vi "Main.vi"() -> ()   [LabVIEW 2017]
uses:
  support/Data Share Type.ctl
  D:/upwork/urartu project/urartu/vs/MapNetControl/bin/Debug/MapNetControl.dll
  vs/MapNetControl/bin/Debug/MapNetControl.dll
panel:
  in  "Add Button":bool
  in  "Longitude, deg:":dbl=27.559764
  in  "Latitude, deg:":dbl=53.907767
  in  "Map folder:":path
  in  "Exit Button":bool
  in  "MapNetControl":refnum<k24>(container)
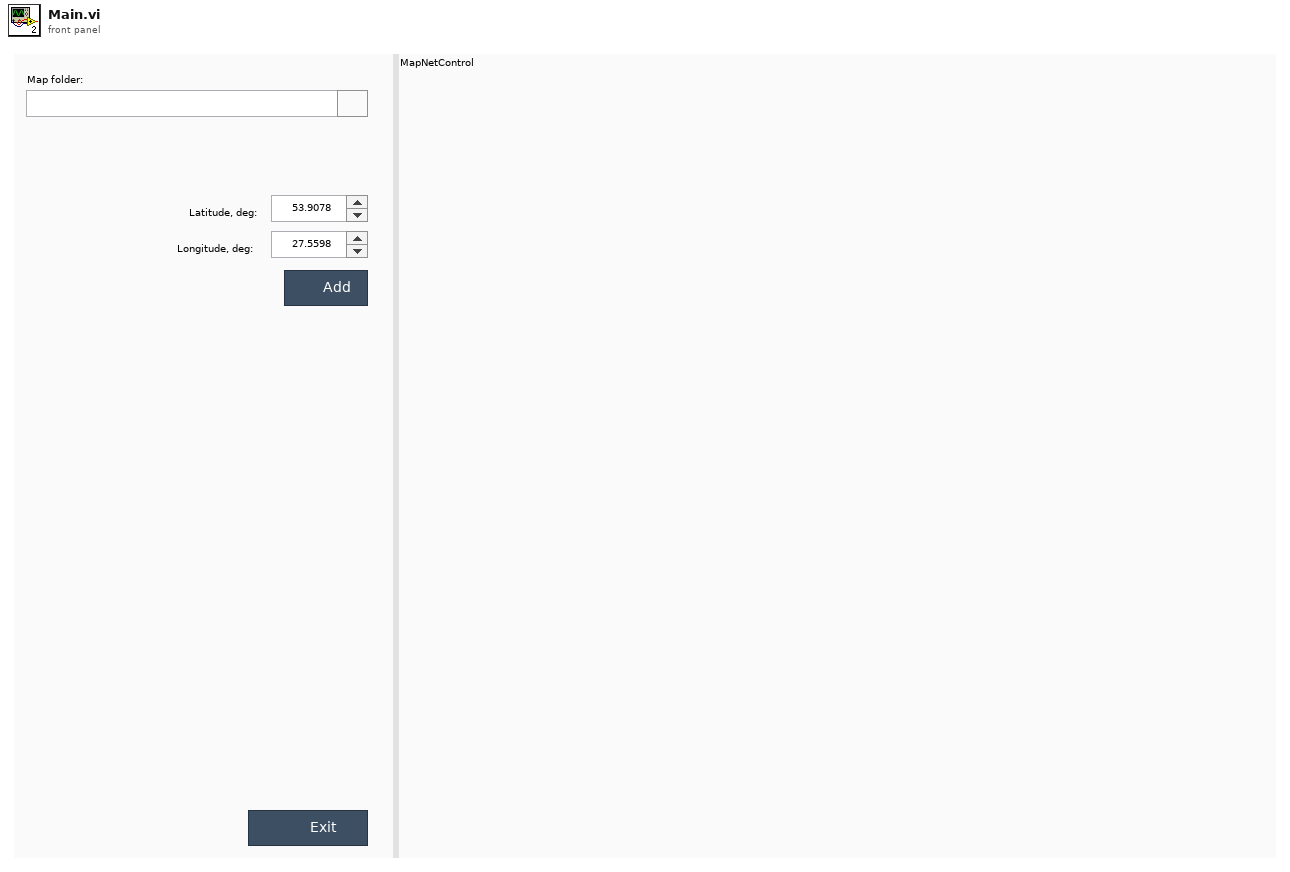
[diagram p1: front panel]
types:
  T1 = typedef "Data Share Type.ctl" = cluster{"Map folder":path, "Latitude, deg:":dbl, "Longitude, deg:":dbl}
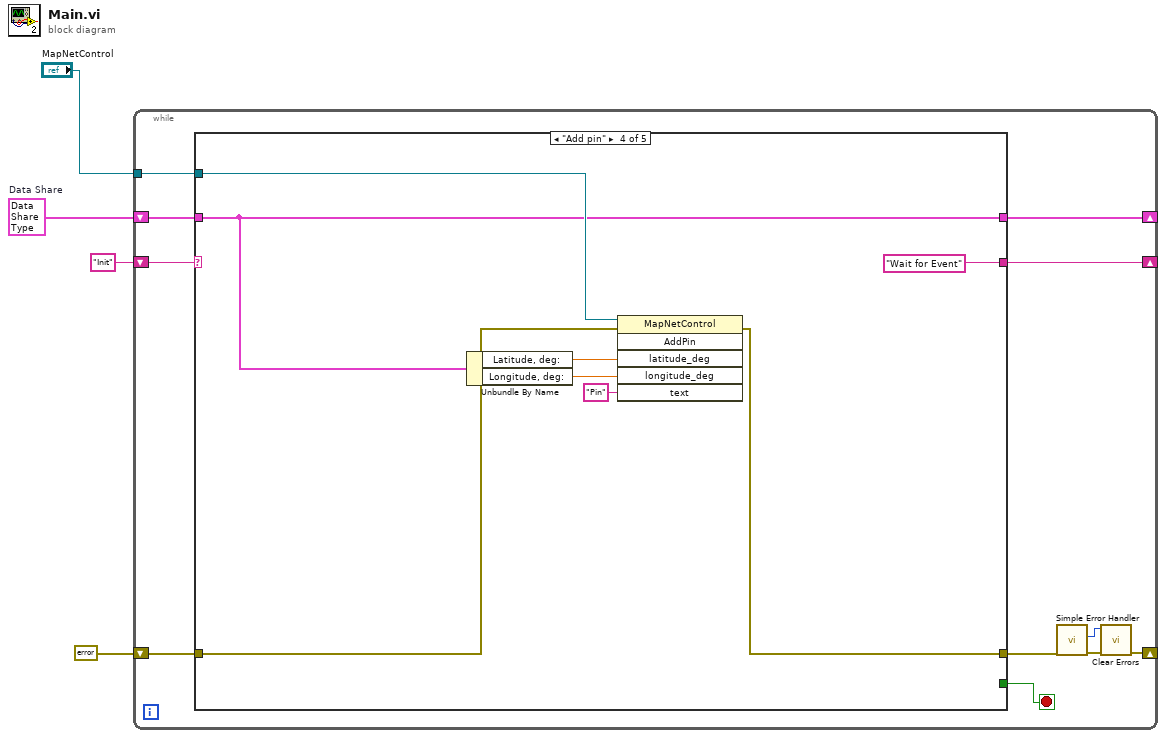
[diagram p0: block diagram]
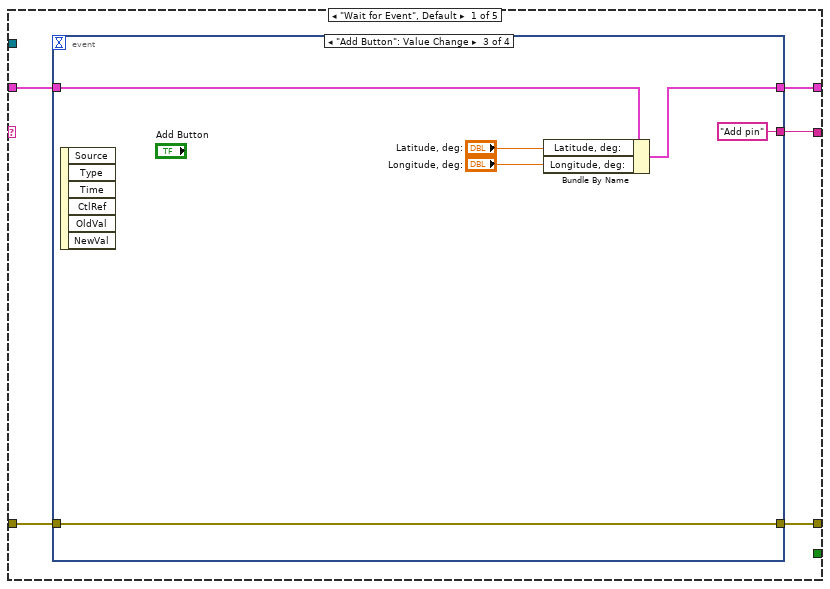
[diagram p2: hidden frame]
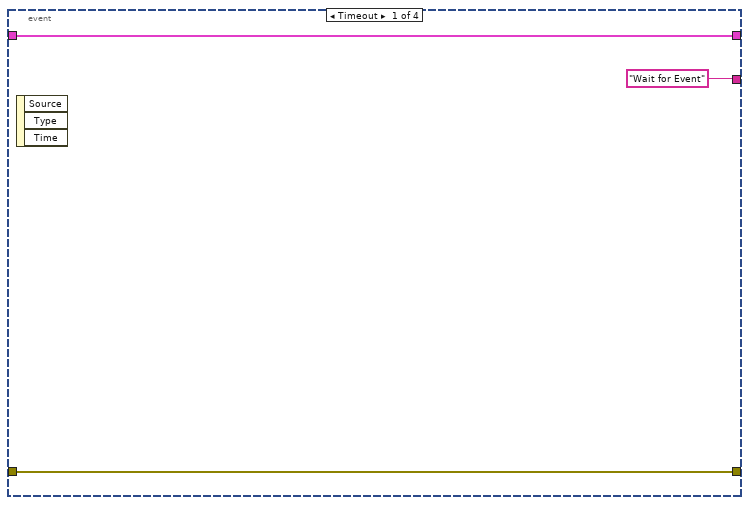
[diagram p3: hidden frame]
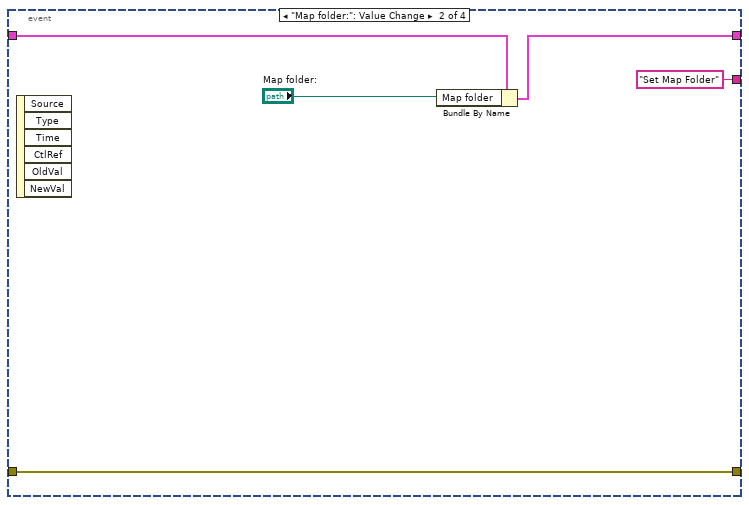
[diagram p4: hidden frame]
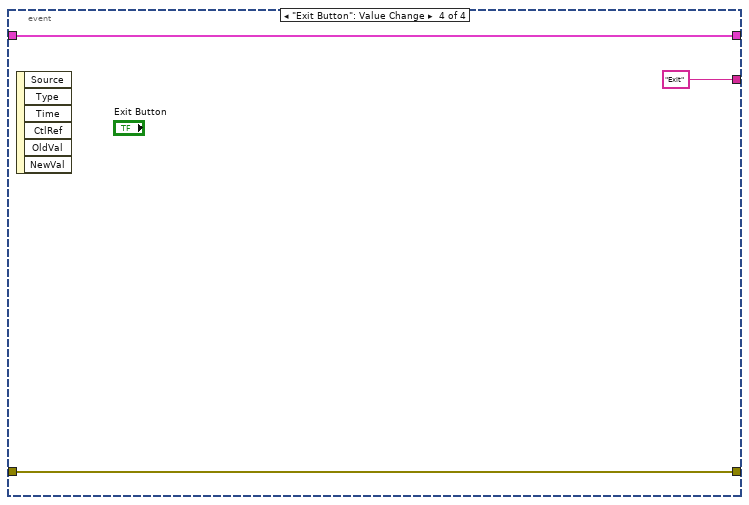
[diagram p5: hidden frame]
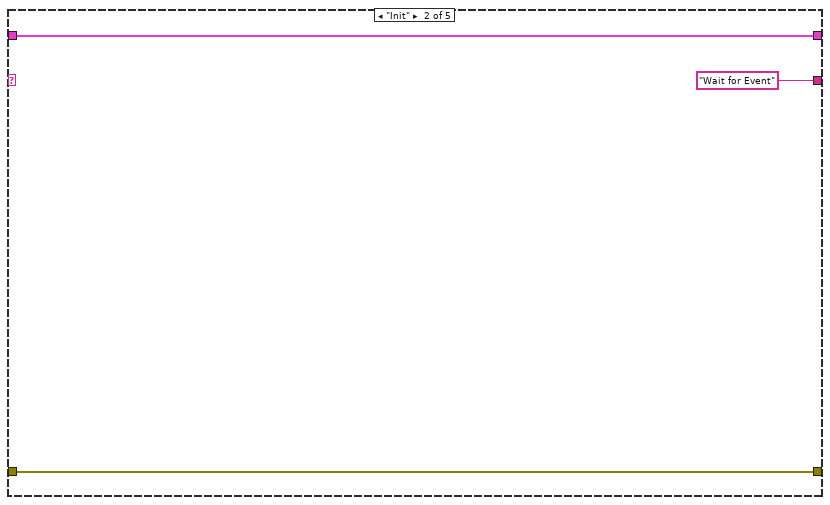
[diagram p6: hidden frame]
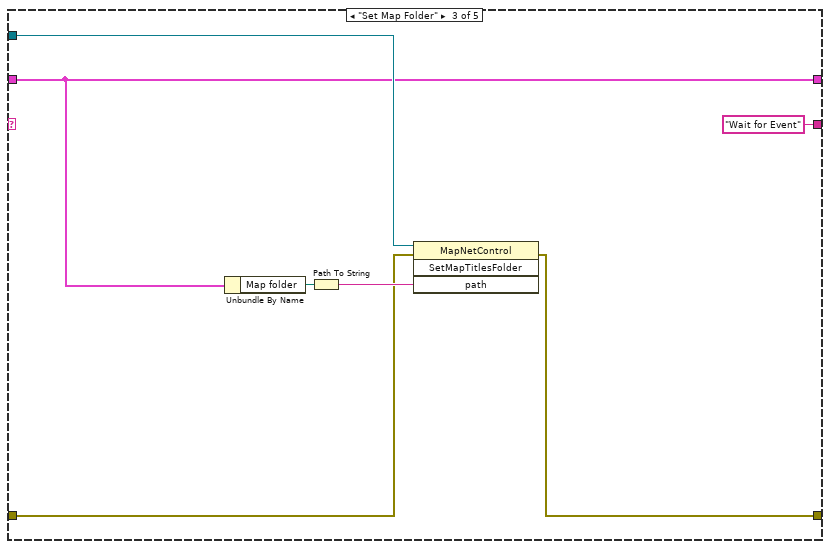
[diagram p7: hidden frame]
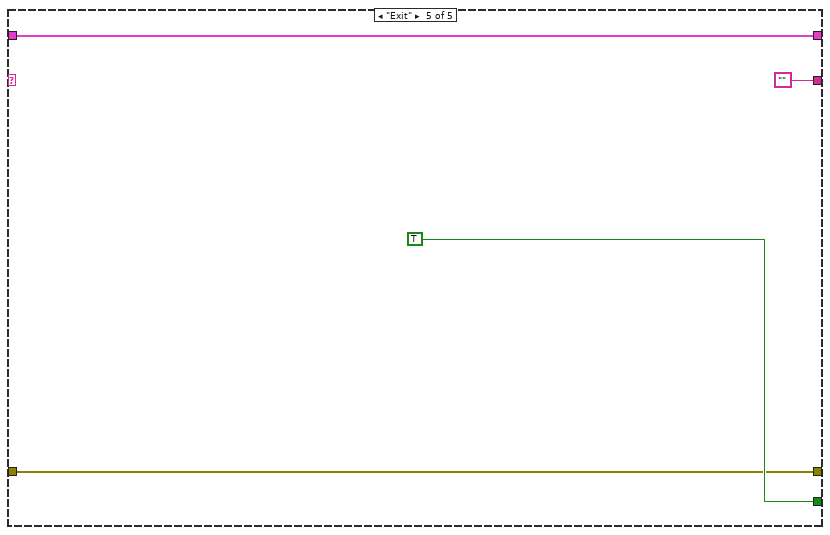
[diagram p8: hidden frame]
diagram:
  w2 = T1 {"Map folder"=path "", "Latitude, deg:"=53.907767, "Longitude, deg:"=27.559764}  # Data Share
  n1 = while {
    tunnel: "MapNetControl" -> [w12]
    shift-right: [w14] -> _
    shift-left: "Init" -> [w15]
    shift-right: [w10] -> _
    shift-left: w2 -> [w11]
    shift-right: [w5] -> _
    shift-left: errorcluster {"status"=FALSE, "code"=0, "source"=""} ("error in (no error)") -> [w9]
    stop <- w13 stop-if-true
    n2 = case shown="\"Add pin\"" w15 {
      tunnel: [w20 "Wait for Event" "Wait for Event" "Wait for Event" ""] -> w14
      tunnel: [_ _ _ _ TRUE] -> w13
      tunnel: w12 -> [_ _ w45 w54 _]
      tunnel: w11 -> [w19 w39 w44 w51 w57]
      tunnel: [w18 w39 w44 w51 w57] -> w10
      tunnel: w9 -> [w17 w38 w42 w53 w56]
      tunnel: [w16 w38 w41 w52 w56] -> w8
      frame "Wait for Event", Default {
        n3 = event shown="[2] \"Add Button\": Value Change" {
          selector: _ -> [_ _ _ _]
          dyn-events: _ -> [_ _ _ _]
          timeout: _ -> [_ _ _ _]
          tunnel: ["Wait for Event" "Set Map Folder" "Add pin" "Exit"] -> w20
          tunnel: [w22 w27 w31 w36] -> w18
          tunnel: w19 -> [w22 w28 w32 w36]
          tunnel: w17 -> [w21 w24 w34 w35]
          tunnel: [w21 w24 w34 w35] -> w16
          event Timeout {
            n4 = event-data() -> ()  [unwired: 1 in, 3 out]
          }
          event "Map folder:": Value Change {
            n5 = event-data() -> ()  [unwired: 1 in, 6 out]
            n6 = Bundle By Name(cluster=w28, "Map folder"="Map folder:") -> (w27:T1)
          }
          event "Add Button": Value Change {
            n7 = event-data() -> ()  [unwired: 1 in, 6 out]
            n8 = Bundle By Name(cluster=w32, "Latitude, deg:"="Latitude, deg:", "Longitude, deg:"="Longitude, deg:") -> (w31:T1)
          }
          event "Exit Button": Value Change {
            n9 = event-data() -> ()  [unwired: 1 in, 6 out]
          }
        }
      }
      frame "Init" {
      }
      frame "Set Map Folder" {
        n10 = Unbundle By Name(w44) -> ("Map folder"=w43:path)
        n11 = Path To String(path=w43) -> (string=w46:string)
        n12 = invoke class="MapNetControl" method="SetMapTitlesFolder"(reference=w45, error in=w42, "path"=w46) -> (error out=w41:errorcluster)  [unwired: 1 in, 3 out]
      }
      frame "Add pin" {
        n13 = Unbundle By Name(w51) -> ("Latitude, deg:"=w50:dbl, "Longitude, deg:"=w49:dbl)
        n14 = invoke class="MapNetControl" method="AddPin"(reference=w54, error in=w53, "latitude_deg"=w50, "longitude_deg"=w49, "text"="Pin") -> (error out=w52:errorcluster)  [unwired: 1 in, 5 out]
      }
      frame "Exit" {
      }
    }
    n15 = call <vilib>:"Simple Error Handler.vi"("error in (no error)"=w8) -> ("code out"=w6:i32, "error out"=w7:errorcluster)  [unwired: 4 in, 3 out]
    n16 = call <vilib>:"Clear Errors.vi"("error in (no error)"=w7, "specific error code to clear (0: all)"=w6) -> ("error out"=w5:errorcluster)  [unwired: 4 in, 1 out]
  }
